vi "ArrayGlobal_CCarga.vi"(0 "Function":T1(ring), 1 "Tiempo":dbl[](array[numeric]) format="%.2f", 2 "Carga":dbl[](array[numeric]) format="%.2f", 3 "LVDT":dbl[](array[numeric]) format="%.2f", 4 "Pres_Poros":dbl[](array[numeric]) format="%.2f", 6 "Path":path) -> (16 "ArrayOut":dbl[](array[numeric]) format="%.2f")   [LabVIEW 2015]
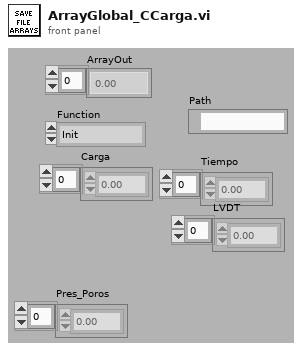
[diagram p1: front panel]
types:
  T1 = enum16{"Init", "Write", "Read array", "Read subarray"}
  T2 = enum16{"open", "open or create", "create or replace", "create", "open (read-only)"}
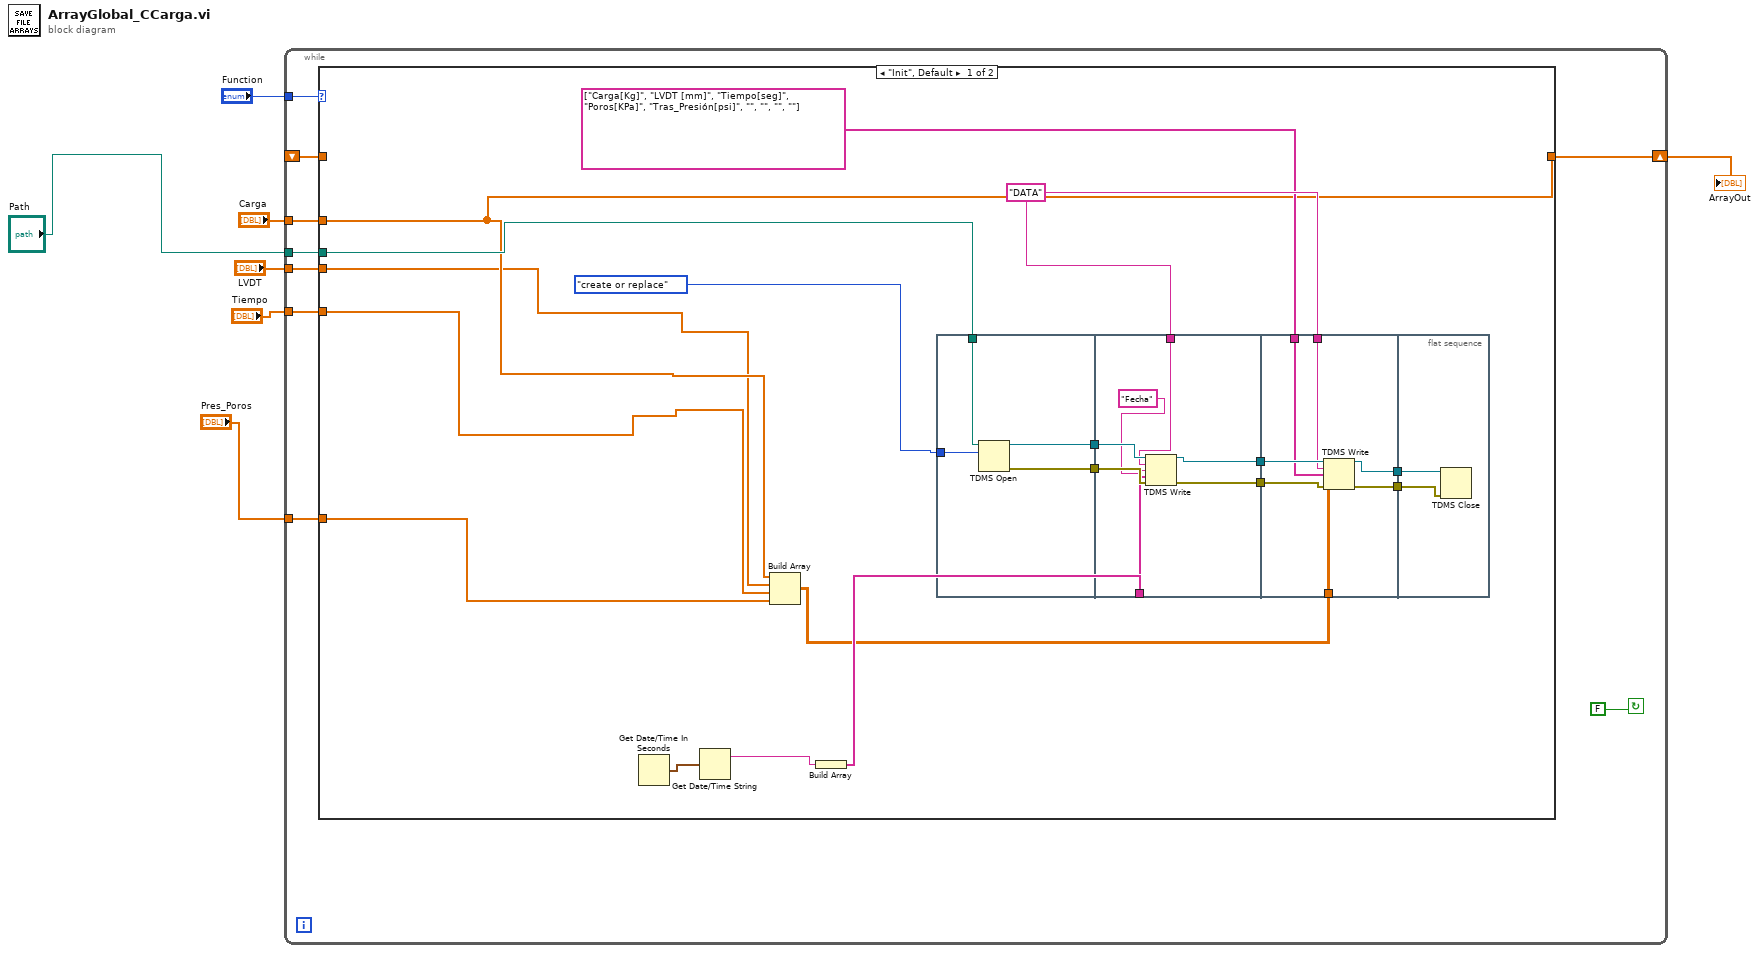
[diagram p0: block diagram]
diagram:
  n1 = while {
    tunnel: "Function" -> [w16]
    shift-right: [w15] -> w5
    shift-left: _ -> [w14]
    tunnel: "Carga" -> [w13]
    tunnel: "LVDT" -> [w11]
    tunnel: "Tiempo" -> [w10]
    tunnel: "Path" -> [w9]
    tunnel: "Pres_Poros" -> [w8]
    stop <- FALSE continue-if-true
    n2 = case shown="\"Init\", Default" w16 {
      tunnel: [w19 w55] -> w15
      tunnel: w14 -> [_ w55]
      tunnel: w13 -> [w19 _]
      tunnel: w11 -> [w18 _]
      tunnel: w10 -> [w21 _]
      tunnel: w9 -> [w22 _]
      tunnel: w8 -> [w17 _]
      frame "Init", Default {
        w26 = "DATA"
        n3 = Get Date/Time In Seconds() -> (seconds since 1Jan1904=w28:timestamp)
        n4 = Get Date/Time String(seconds (now)=w28) -> (date string=w23:string)  [unwired: 2 in, 1 out]
        n5 = Build Array(w19, w18, w21, w17) -> (w20:dbl[][])
        n6 = Build Array(w23) -> (w27:string[])
        n7 = flat-sequence {
          tunnel: T2."create or replace" ("operation (0:open)") -> [w38]
          tunnel: w22 -> [w37]
          tunnel: [w36] -> w34
          tunnel: [w35] -> w33
          tunnel: w34 -> [w45]
          tunnel: w33 -> [w44]
          tunnel: [w43] -> w32
          tunnel: [w42] -> w31
          tunnel: w26 -> [w40]
          tunnel: w27 -> [w39]
          tunnel: w32 -> [w52]
          tunnel: [w51] -> w30
          tunnel: [w50] -> w29
          tunnel: w31 -> [w49]
          tunnel: w26 -> [w48]
          tunnel: string[] ["Carga[Kg]", "LVDT [mm]", "Tiempo[seg]", "Poros[KPa]", "Tras_Presión[psi]", "", "", "", ""] ("channel name(s) in (Untitled)") -> [w47]
          tunnel: w20 -> [w46]
          tunnel: w30 -> [w54]
          tunnel: w29 -> [w53]
          frame #0 {
            n8 = TDMS Open(10:w38, 11:w37) -> (0:w35:errorcluster, 3:w36:refnum<k34>)  [unwired: 5 in]
          }
          frame #1 {
            n9 = TDMS Write(0:w45, 5:w40, 7:"Fecha" ("channel name(s) in (Untitled)"), 9:w39, 11:w44) -> (4:w43:refnum<k34>, 15:w42:errorcluster)  [unwired: 1 in, 2 out]
          }
          frame #2 {
            n10 = TDMS Write(0:w52, 5:w48, 7:w47, 9:w46, 11:w49) -> (4:w51:refnum<k34>, 15:w50:errorcluster)  [unwired: 1 in, 2 out]
          }
          frame #3 {
            n11 = TDMS Close(8:w53, 11:w54) -> ()  [unwired: 2 out]
          }
        }
      }
      frame "Read array" {
      }
    }
  }
  "ArrayOut" <- w5
